vi "Fbeta_Score.vi"(6 "Type y_pred":T1(ring), 7 "Type y_true":T1(ring), 8 "error in (no error)":errorcluster caption="entrée d'erreur (pas d'erreur)", 9 "y_pred":string[][](array[string]), 10 "y_true":string[][](array[string]), 11 "fbeta_score":T3={"beta"=0.0, "labels"=[], "pos_label"={"dtype_pos_label"="int", "pos_label"="1"}, "average"="binary", "sample_weight"=[], "zero_division"={"dtype_zero_division"="str", "zero_division"="warn"}}) -> (0 "error out":errorcluster caption="sortie d'erreur", 3 "Data":T2)   [LabVIEW 2020]
doc: "Compute the F-beta score\n\nThe F-beta score is the weighted harmonic mean of precision and recall, reaching its optimal value at 1 and its worst value at 0.\n\nThe beta parameter determines the weight of recall in the combined score. beta < 1 lends more weight to precision, while beta > 1 favors recall (beta -> 0 considers only precision, beta -> +inf only recall).\n\n\n\nParameters : \n\n- y_true : 1d array-like, or label indicator array / sparse matrix\nGround truth (correct) target values.\n\n- y_pred : 1d array-like, or label indicator array / sparse matrix\nEstimated targets as returned by a classifier.\n\n- beta : float\nDetermines the weight of recall in the combined score.\n\n- labels : list, optional\nThe set of labels to include when average != 'binary', and their order if average is None. Labels present in the data can be excluded, for example to calculate a multiclass average ignoring a majority negative class, while labels not present in the data will result in 0 components in a macro average. For multilabel targets, labels are column indices. By default, all labels in y_true and y_pred are used in sorted order.\n\n- pos_label : str or int, 1 by default\nThe class to report if average='binary' and the data is binary. If the data are multiclass or multilabel, this will be ignored; setting labels=[pos_label] and average != 'binary' will report scores for that label only.\n\n- average : string, [None, ‘binary’ (default), ‘micro’, ‘macro’, ‘samples’, ‘weighted’]\nThis parameter is required for multiclass/multilabel targets. If None, the scores for each class are returned. Otherwise, this determines the type of averaging performed on the data:\n\n'binary':\nOnly report results for the class specified by pos_label. This is applicable only if targets (y_{true,pred}) are binary.\n\n'micro':\nCalculate metrics globally by counting the total true positives, false negatives and false positives.\n\n'macro':\nCalculate metrics for each label, and find their unweighted mean. This does not take label imbalance into account.\n\n'weighted':\nCalculate metrics for each label, and find their average weighted by support (the number of true instances for each label). This alters ‘macro’ to account for label imbalance; it can result in an F-score that is not between precision and recall.\n\n'samples':\nCalculate metrics for each instance, and find their average (only meaningful for multilabel classification where this differs from accuracy_score).\n\n- sample_weight : array-like of shape (n_samples,), default=None\nSample weights.\n\n- zero_division : “warn”, 0 or 1, default=”warn”\nSets the value to return when there is a zero division, i.e. when all predictions and labels are negative. If set to “warn”, this acts as 0, but warnings are also raised.\n\nReturns : \n\n- fbeta_score : float (if average is not None) or array of float, shape = [n_unique_labels]\nF-beta score of the positive class in binary classification or weighted average of the F-beta score of each class for the multiclass task."
uses:
  Fbeta_Score.lvclass
panel:
  out "Fbeta_Score.lvclass":refnum<class "Fbeta_Score.lvclass">
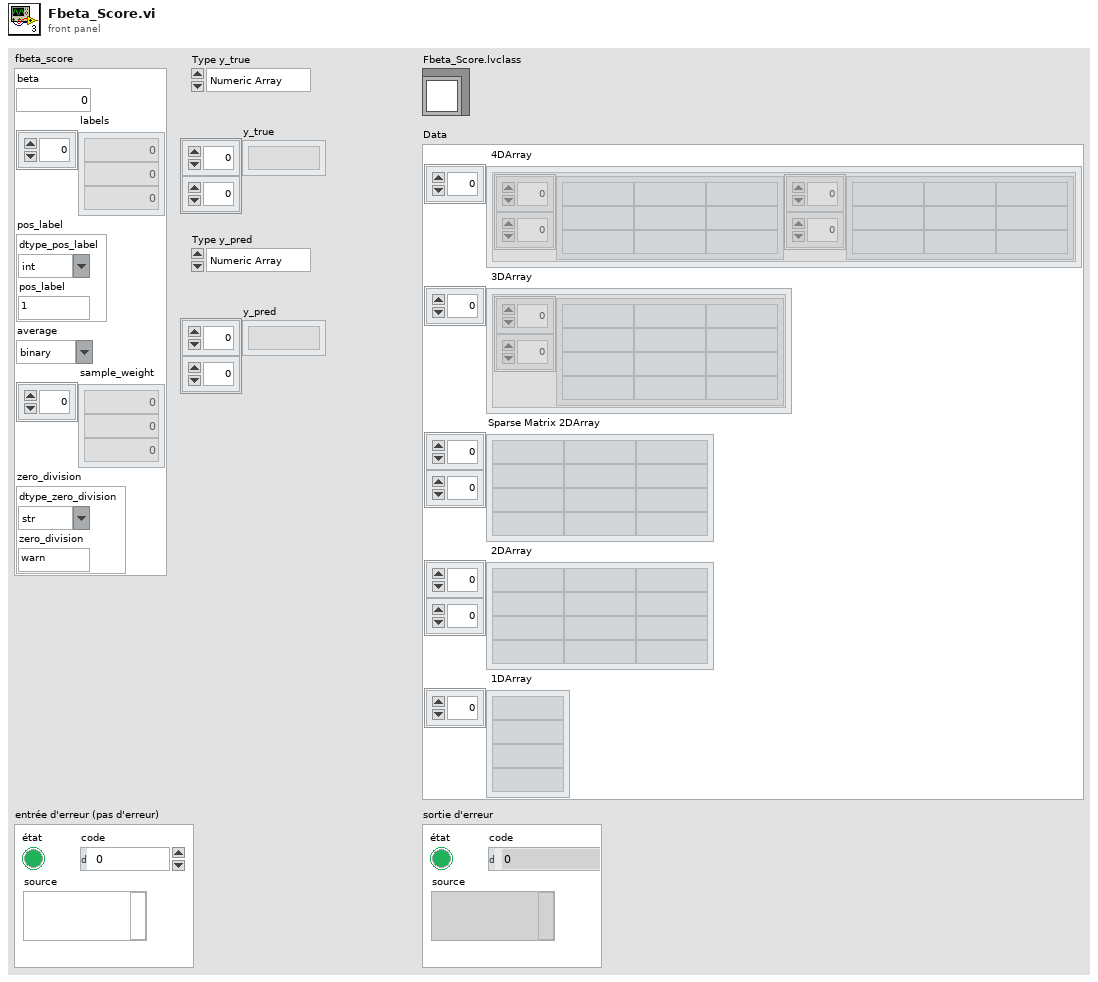
[diagram p1: front panel]
types:
  T1 = enum16{"Numeric Array", "String Array", "Sparse"}
  T2 = cluster{" 4DArray":cluster{"1":string[][], "2":string[][]}[], " 3DArray":cluster{"Tableau":string[][]}[], "Sparse Matrix 2DArray":string[][], " 2DArray":string[][], " 1DArray":string[]}
  T3 = cluster{"beta":dbl, "labels":i32[], "pos_label":cluster{"dtype_pos_label":string, "pos_label":string}, "average":string, "sample_weight":dbl[], "zero_division":cluster{"dtype_zero_division":string, "zero_division":string}}
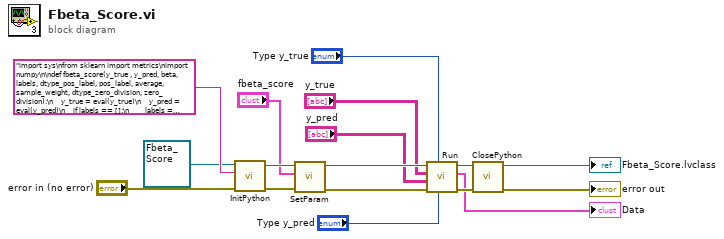
[diagram p0: block diagram]
diagram:
  n1 = call-dynamic "InitPython.vi"("error in (no error)"="error in (no error)", "Python Instruction"="import sys\nfrom sklearn import metrics\nimport numpy\n\ndef fbeta_score(y_true , y_pred, beta, labels, dtype_pos_label, pos_label, average, sample_weight, dtype_zero_division, zero_division):\n    y_true = eval(y_true)\n    y_pred = eval(y_pred)\n    if labels == []:\n        labels = None\n    if dtype_pos_label == 'int':\n        pos_label = eval(pos_label)\n    if average == 'None':\n        average = None\n    if sample_weight == []:\n        sample_weight = None\n    if dtype_zero_division == 'int':\n        zero_division = eval(zero_division)\n    try:\n        fbeta_score = metrics.fbeta_score(y_true , y_pred, beta, labels, pos_label, average, sample_weight, zero_division)\n        fbeta_score = fbeta_score.tolist()\n        return str(fbeta_score)\n    except:\n        erreur = sys.exc_info()\n        typerr = u\"%s\" % (erreur[0])\n        typerr = typerr[typerr.find(\"'\")+1:typerr.rfind(\"'\")]\n        msgerr = u\"%s\" % (erreur[1])\n        message = str('/!\\\\ {0} : {1}'. format(typerr,msgerr))\n        return message", "Scikit-learn en entrée"=refnum<class "Fbeta_Score.lvclass"> refnum ("Fbeta_Score.lvclass")) -> ("error out"=w15:errorcluster, "Scikit-learn en sortie"=w14:refnum<class "Fbeta_Score.lvclass">)  [unwired: 7 in]
  n2 = call-dynamic "SetParam.vi"("error in (no error)"=w15, "fbeta_score"="fbeta_score", "Fbeta_Score.lvclass"=w14) -> ("error out"=w11:errorcluster, "Fbeta_Score.lvclass"=w10:refnum<class "Fbeta_Score.lvclass">)  [unwired: 7 in]
  n3 = call-dynamic "Run.vi"("Type y_pred"="Type y_pred", "Type y_true"="Type y_true", "error in (no error)"=w11, "y_pred"="y_pred", "y_true"="y_true", "Fbeta_Score.lvclass"=w10) -> ("error out"=w9:errorcluster, "Data"=→"Data":T2, "Fbeta_Score.lvclass"=w8:refnum<class "Fbeta_Score.lvclass">)  [unwired: 3 in]
  n4 = call-dynamic "ClosePython.vi"("error in (no error)"=w9, "Scikit-learn en entrée"=w8) -> ("error out"=→"error out":errorcluster, "Scikit-learn en sortie"=→"Fbeta_Score.lvclass":refnum<class "Fbeta_Score.lvclass">)  [unwired: 8 in]
